vi "while_v0_v2.vi"() -> ()   [LabVIEW 2009]
panel:
  in  "stop":bool
  out "Numeric":dbl
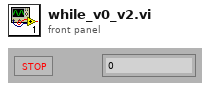
[diagram p1: front panel]
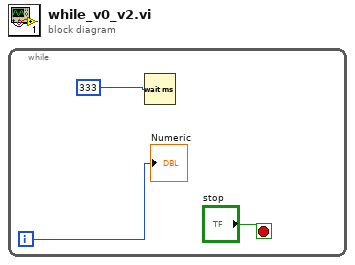
[diagram p0: block diagram]
diagram:
  n1 = while {
    i -> [w1]
    stop <- "stop" stop-if-true
    n2 = Wait (ms)(milliseconds to wait=333) -> ()  [unwired: 1 out]
    "Numeric" <- w1
  }
